vi "Host_Reader.vi"() -> ()   [LabVIEW 2021]
uses:
  Model_Updating_Classes/DROPBEAR_Model_Updating/DROPBEAR_Model_Updating.lvclass
panel:
  out "Progress":u8(slide) scale=0.0..1000.0
  in  "Tab Control":enum32{"Page 1", "Page 2"}(tab)
  out "Elasped Time (HH:MM:SS)":string caption="Result"
  out "Average Cycle Time (ms)":dbl
  out "StatisticsTime cost":T1
  out "Cycle Time cost":T1
  out "State KF Time cost":T1
  out "FEA Time cost":T1
  out "Sampling Time cost":T1
  out "FFT KF Time cost":T1
  out "FFT Time cost":T1
  out "DAQ Time cost":T1
  out "Signal Quality Stats Position":T2
  out "Signal Quality Stats Frequency":T2
  out "Online Time (HH:MM:SS)":string caption="Result"
  out "Preprocessing Time (HH:MM:SS)":string caption="Result"
  out "Total time":dbl[](array[numeric])
  out "Preprocess time":dbl[](array[numeric])
  out "Online time":dbl[](array[numeric])
  out "Frequency":dynamicdata(graph)
  out "Meter":dynamicdata(graph)
  out "Nodal":dynamicdata(graph)
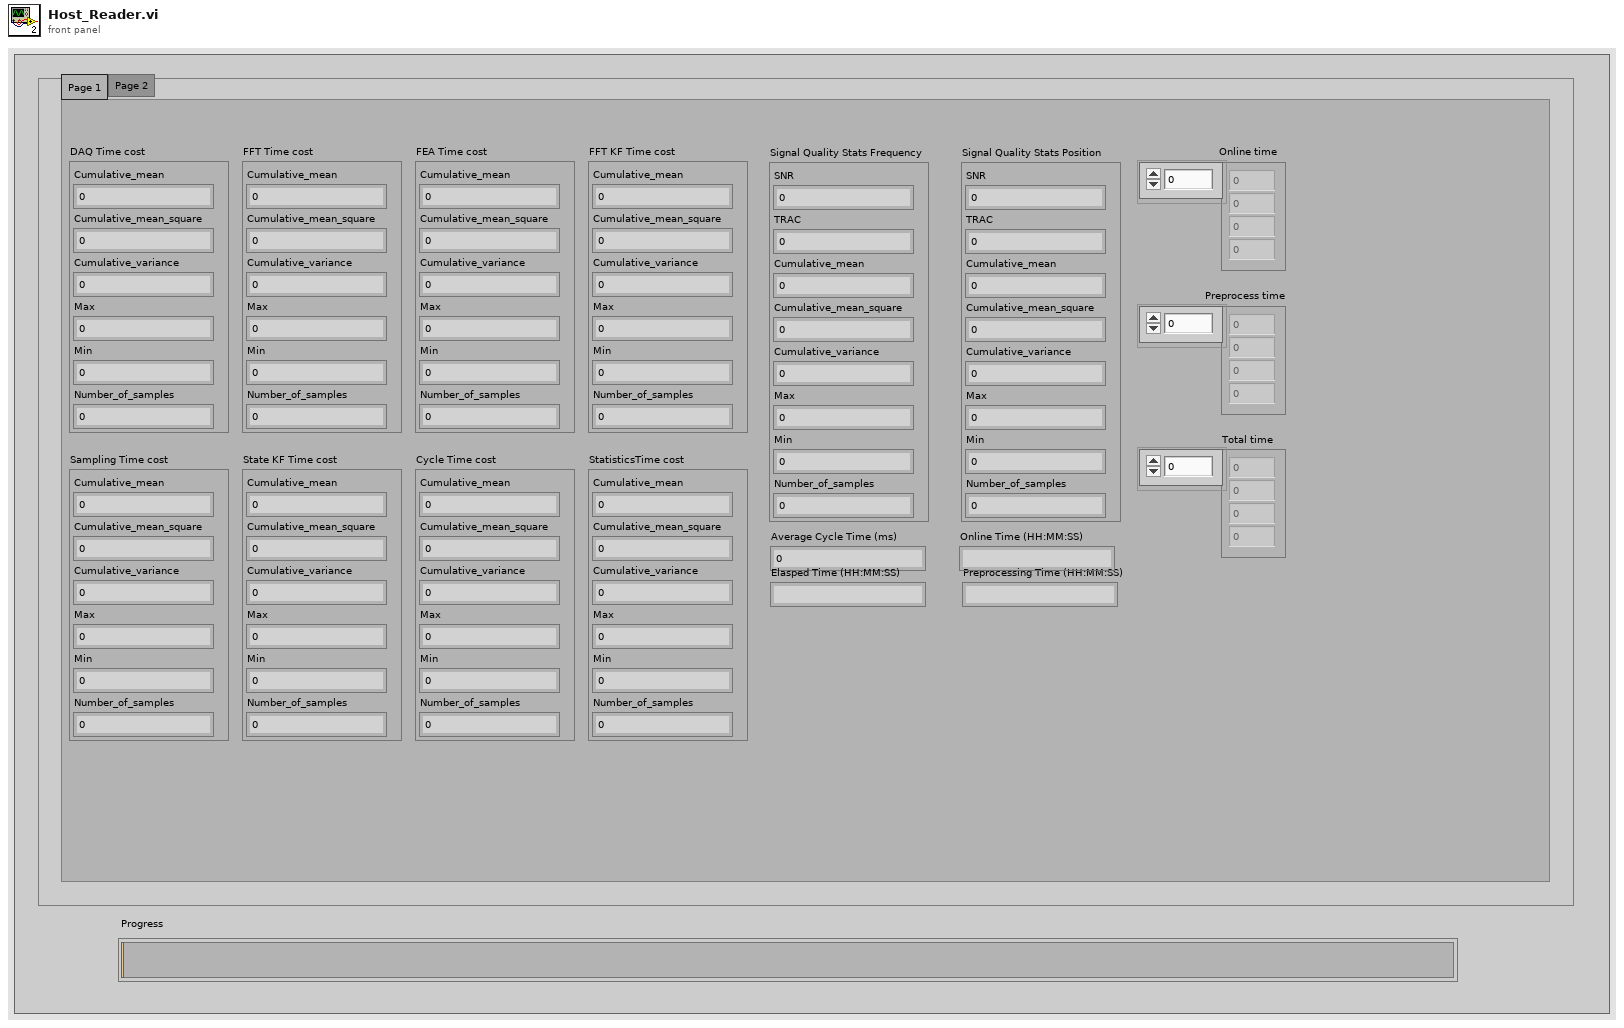
[diagram p1: front panel]
types:
  T1 = cluster{"Cumulative_mean":dbl, "Cumulative_mean_square ":dbl, "Cumulative_variance":dbl, "Max":dbl, "Min":dbl, "Number_of_samples":i32}
  T2 = cluster{"SNR":dbl, "TRAC":dbl, "Cumulative_mean":dbl, "Cumulative_mean_square ":dbl, "Cumulative_variance":dbl, "Max":dbl, "Min":dbl, "Number_of_samples":i32}
  T3 = cluster{"Signal Quality Stats Frequency":cluster{"SNR":dbl, "TRAC":dbl, "Cumulative_mean":dbl, "Cumulative_mean_square ":dbl, "Cumulative_variance":dbl, "Max":dbl, "Min":dbl, "Number_of_samples":i32}, "Signal Quality Stats Position":cluster{"SNR":dbl, "TRAC":dbl, "Cumulative_mean":dbl, "Cumulative_mean_square ":dbl, "Cumulative_variance":dbl, "Max":dbl, "Min":dbl, "Number_of_samples":i32}}
  T4 = cluster{"DAQ Time cost":cluster{"Cumulative_mean":dbl, "Cumulative_mean_square ":dbl, "Cumulative_variance":dbl, "Max":dbl, "Min":dbl, "Number_of_samples":i32}, "FFT Time cost":cluster{"Cumulative_mean":dbl, "Cumulative_mean_square ":dbl, "Cumulative_variance":dbl, "Max":dbl, "Min":dbl, "Number_of_samples":i32}, "FFT KF Time cost":cluster{"Cumulative_mean":dbl, "Cumulative_mean_square ":dbl, "Cumulative_variance":dbl, "Max":dbl, "Min":dbl, "Number_of_samples":i32}, "Sampling Time cost":cluster{"Cumulative_mean":dbl, "Cumulative_mean_square ":dbl, "Cumulative_variance":dbl, "Max":dbl, "Min":dbl, "Number_of_samples":i32}, "FEA Time cost":cluster{"Cumulative_mean":dbl, "Cumulative_mean_square ":dbl, "Cumulative_variance":dbl, "Max":dbl, "Min":dbl, "Number_of_samples":i32}, "State KF Time cost":cluster{"Cumulative_mean":dbl, "Cumulative_mean_square ":dbl, "Cumulative_variance":dbl, "Max":dbl, "Min":dbl, "Number_of_samples":i32}, "Cycle Time cost":cluster{"Cumulative_mean":dbl, "Cumulative_mean_square ":dbl, "Cumulative_variance":dbl, "Max":dbl, "Min":dbl, "Number_of_samples":i32}, "StatisticsTime cost":cluster{"Cumulative_mean":dbl, "Cumulative_mean_square ":dbl, "Cumulative_variance":dbl, "Max":dbl, "Min":dbl, "Number_of_samples":i32}}
  T5 = cluster{"Frequency":dynamicdata, "Meters":dynamicdata, "Nodal":dynamicdata}
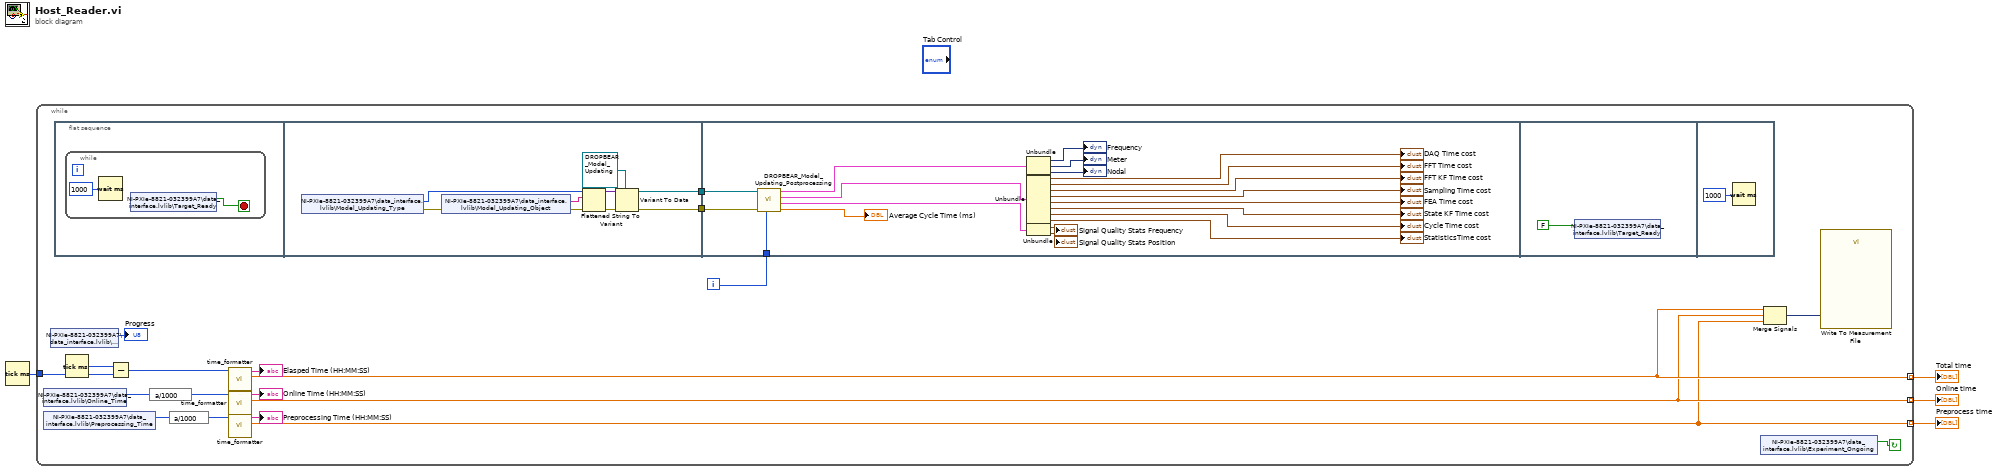
[diagram p0: block diagram]
diagram:
  n1 = Tick Count (ms)() -> (millisecond timer value=w4:u32)
  n2 = while {
    tunnel: w4 -> [w22]
    tunnel: [w10] -> w3 mode=indexing
    tunnel: [w9] -> w1 mode=indexing
    tunnel: [w8] -> w2 mode=indexing
    i -> [w6]
    stop <- w19 continue-if-true
    n3 = shared-variable "NI-PXIe-8821-032399A7\\data_interface.lvlib\\Online_Time"() -> (w5:u64)  [unwired: 1 in, 1 out]
    n4 = shared-variable "NI-PXIe-8821-032399A7\\data_interface.lvlib\\Preprocessing_Time"() -> (w15:i64)  [unwired: 1 in, 1 out]
    n5 = shared-variable "NI-PXIe-8821-032399A7\\data_interface.lvlib\\Progress"() -> (→"Progress":i8)  [unwired: 1 in, 1 out]
    n6 = flat-sequence {
      tunnel: [w27] -> w21
      tunnel: [w26] -> w20
      tunnel: w21 -> [w37]
      tunnel: w20 -> [w36]
      tunnel: w6 -> [w35]
      frame #0 {
        n7 = while {
          stop <- w25 stop-if-true
          n8 = Wait (ms)(milliseconds to wait=u32 1000) -> ()  [unwired: 1 out]
          n9 = shared-variable "NI-PXIe-8821-032399A7\\data_interface.lvlib\\Target_Ready"() -> (w25:bool)  [unwired: 1 in, 1 out]
        }
      }
      frame #1 {
        n10 = shared-variable "NI-PXIe-8821-032399A7\\data_interface.lvlib\\Model_Updating_Type"() -> (w31:i16[], error out=w34:errorcluster)  [unwired: 1 in]
        n11 = shared-variable "NI-PXIe-8821-032399A7\\data_interface.lvlib\\Model_Updating_Object"(error in=w34) -> (w32:string, error out=w33:errorcluster)
        n12 = Flattened String To Variant(4:w33, 6:w32, 7:w31) -> (0:w28:errorcluster, 3:w29:variant)
        n13 = Variant To Data(error in=w28, type=refnum<class "DROPBEAR_Model_Updating.lvclass"> refnum ("DROPBEAR_Model_Updating.lvclass"), Variant=w29) -> (data=w27:refnum<class "DROPBEAR_Model_Updating.lvclass">, error out=w26:errorcluster)
      }
      frame #2 {
        n14 = call "DROPBEAR_Model_Updating_Postprocessing.vi"("Test number"=w35, "error in (no error)"=w36, "DROPBEAR_Model_Updating in"=w37) -> ("Cycle time (ms)"=→"Average Cycle Time (ms)":dbl, "Signal Quality"=w54:T3, "Timing stats"=w51:T4, "Plots"=w42:T5)  [unwired: 5 in]
        n15 = Unbundle(w42) -> ("Frequency"=→"Frequency":dynamicdata, "Meters"=→"Meter":dynamicdata, "Nodal"=→"Nodal":dynamicdata)
        n16 = Unbundle(w51) -> ("DAQ Time cost"=→"DAQ Time cost":T1, "FFT Time cost"=→"FFT Time cost":T1, "FFT KF Time cost"=→"FFT KF Time cost":T1, "Sampling Time cost"=→"Sampling Time cost":T1, "FEA Time cost"=→"FEA Time cost":T1, "State KF Time cost"=→"State KF Time cost":T1, "Cycle Time cost"=→"Cycle Time cost":T1, "StatisticsTime cost"=→"StatisticsTime cost":T1)
        n17 = Unbundle(w54) -> ("Signal Quality Stats Frequency"=→"Signal Quality Stats Frequency":T2, "Signal Quality Stats Position"=→"Signal Quality Stats Position":T2)
      }
      frame #3 {
        n18 = shared-variable "NI-PXIe-8821-032399A7\\data_interface.lvlib\\Target_Ready"(FALSE ("Process_Halt")) -> ()  [unwired: 1 in, 1 out]
      }
      frame #4 {
        n19 = Wait (ms)(milliseconds to wait=u32 1000) -> ()  [unwired: 1 out]
      }
    }
    n20 = Tick Count (ms)() -> (millisecond timer value=w23:u32)
    n21 = Subtract(x=w23, y=w22) -> (x-y=w17:u32)
    n22 = expression code="a/1000"(w5) -> (w13:u64)
    n23 = expression code="a/1000"(w15) -> (w14:i64)
    n24 = call "time_formatter.vi"("time (ms)"=w17) -> ("time (sec)"=w10:dbl, "Elasped Time (HH:MM:SS)"=→"Elasped Time (HH:MM:SS)":string)  [unwired: 9 in]
    n25 = call "time_formatter.vi"("time (ms)"=w13) -> ("time (sec)"=w9:dbl, "Elasped Time (HH:MM:SS)"=→"Online Time (HH:MM:SS)":string)  [unwired: 9 in]
    n26 = call "time_formatter.vi"("time (ms)"=w14) -> ("time (sec)"=w8:dbl, "Elasped Time (HH:MM:SS)"=→"Preprocessing Time (HH:MM:SS)":string)  [unwired: 9 in]
    n27 = shared-variable "NI-PXIe-8821-032399A7\\data_interface.lvlib\\Experiment_Ongoing"() -> (w19:bool)  [unwired: 1 in, 1 out]
    n28 = Merge Signals(w10, w9, w8) -> (w7:dynamicdata)
    n29 = call "Write To Measurement File"("Signals"=w7) -> ()  [unwired: 16 in, 3 out]
  }
  "Total time" <- w3
  "Preprocess time" <- w2
  "Online time" <- w1
